vi "Keithley2400x2.vi"() -> ()   [LabVIEW 2014]
uses:
  <vilib>/Utility/file.llb/Write To Spreadsheet File (string).vi
panel:
  in  "stop":bool
  in  "Source Mode  (0: Voltage)":u16(ring) items=["Voltage", "Current"]
  in  "VISA resource name 2":refnum<visa-resource-name>
  in  "Serial Configuration":T1={"Baud Rate"=9600, "Parity"=0, "Data Bits"=8, "Stop Bits"=10, "Flow Control"=0} {"Flow Control" items=["None", "XON/XOFF", "RTS/CTS", "XON/XOFF & RTS/CTS", "DTR/DSR", "XON/XOFF & DTR/DSR"]; "Stop Bits" items=["1.0"=10, "1.5"=15, "2.0"=20]; "Data Bits" items=["7"=7, "8"=8]; "Parity" items=["None", "Odd", "Even", "Mark", "Space"]; "Baud Rate" items=["300"=300, "600"=600, "1200"=1200, "2400"=2400, "4800"=4800, "9600"=9600, "19200"=19200]}
  in  "Файл записи замеров":path
  in  "Ограничение":dbl format="%.2f"
  out "Замер":string
  in  "Выход":dbl
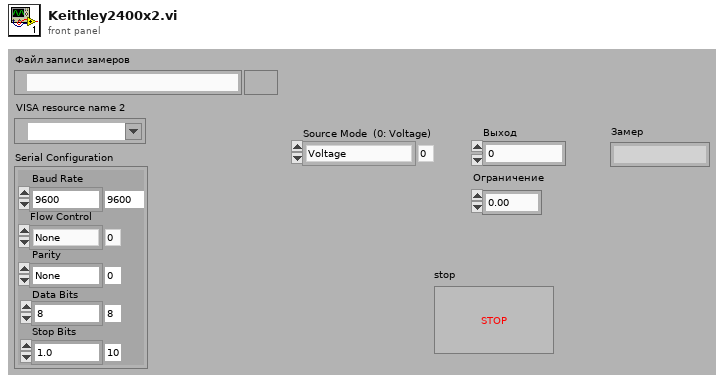
[diagram p1: front panel]
types:
  T1 = cluster{"Baud Rate":u32, "Parity":u16, "Data Bits":u16, "Stop Bits":u16, "Flow Control":u16}
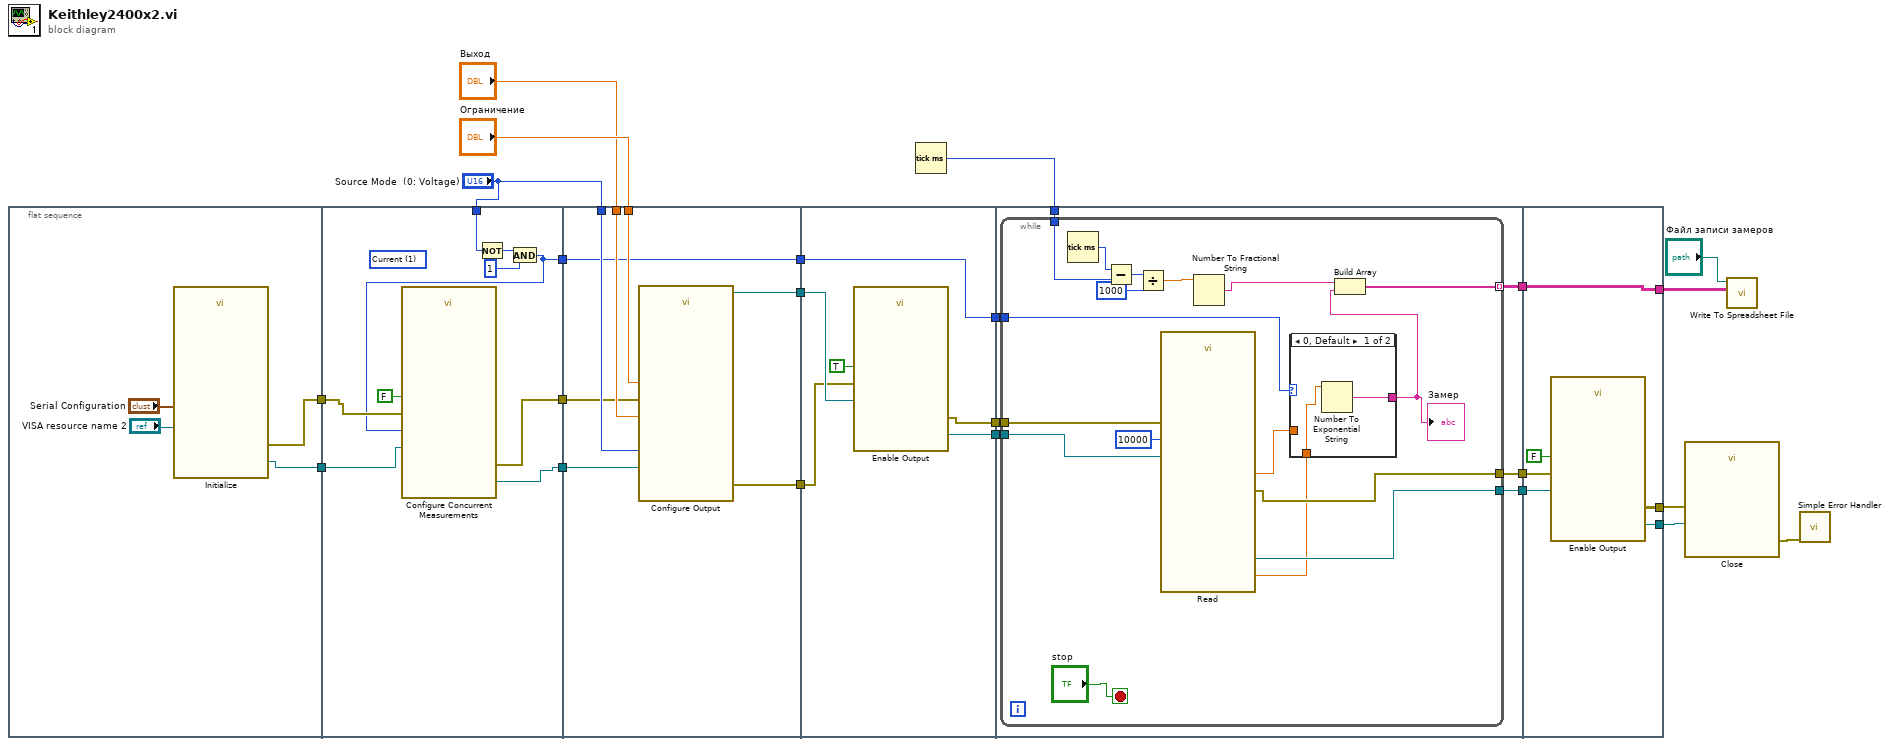
[diagram p0: block diagram]
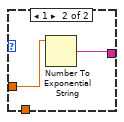
[diagram p2: hidden frame]
diagram:
  n1 = flat-sequence {
    tunnel: [w25] -> w8
    tunnel: [w24] -> w6
    tunnel: w8 -> [w34]
    tunnel: [w35] -> w7
    tunnel: w6 -> [w33]
    tunnel: [w36] -> w5
    tunnel: "Source Mode  (0: Voltage)" -> [w31]
    tunnel: [w28] -> w1
    tunnel: "Ограничение" -> [w44]
    tunnel: "Выход" -> [w43]
    tunnel: "Source Mode  (0: Voltage)" -> [w42]
    tunnel: w7 -> [w41]
    tunnel: w5 -> [w40]
    tunnel: [w39] -> w21
    tunnel: [w38] -> w20
    tunnel: [w37] -> w3
    tunnel: w1 -> [w37]
    tunnel: w21 -> [w50]
    tunnel: w20 -> [w49]
    tunnel: [w47] -> w19
    tunnel: [w46] -> w18
    tunnel: w3 -> [w45]
    tunnel: [w45] -> w2
    tunnel: w19 -> [w57]
    tunnel: w18 -> [w56]
    tunnel: w17 -> [w55]
    tunnel: [w54] -> w14
    tunnel: [w53] -> w13
    tunnel: [w52] -> w12
    tunnel: w2 -> [w51]
    tunnel: [w84] -> w15
    tunnel: w14 -> [w84]
    tunnel: w13 -> [w82]
    tunnel: w12 -> [w81]
    tunnel: [w80] -> w11
    tunnel: [w79] -> w10
    frame #0 {
      n2 = call "Initialize.vi"("Serial Configuration"="Serial Configuration", "VISA resource name"="VISA resource name 2") -> ("error out"=w24:errorcluster, "VISA resource name out"=w25:refnum<visa-resource-name>)  [unwired: 8 in]
    }
    frame #1 {
      (unwired) u16 1 items=["Volts", "Current", "Resistance", "Volt, Current", "Volts, Resistance", "Current, Resistance", "All"] ("Measurement Selection (3: Volts, Current)")
      n3 = Not(x=w31) -> (.not. x?=w30:u16)
      n4 = And(x=w30, y=u16 1) -> (x .and. y?=w28:u16)
      n5 = call "Configure Concurrent Measurements.vi"("error in (no error)"=w33, "Measurement Selection (3: Volts, Current)"=w28, "Enable Concurrent Measurements (F: Disable)"=FALSE, "VISA resource name"=w34) -> ("error out"=w36:errorcluster, "VISA resource name out"=w35:refnum<visa-resource-name>)  [unwired: 6 in]
    }
    frame #2 {
      n6 = call "Configure Output.vi"("Source Mode  (0: Voltage)"=w42, "error in (no error)"=w40, "Compliance  Level (0.1)"=w44, "Output Level (0)"=w43, "VISA resource name"=w41) -> ("error out"=w38:errorcluster, "VISA resource name out"=w39:refnum<visa-resource-name>)  [unwired: 5 in]
    }
    frame #3 {
      n7 = call "Enable Output.vi"("error in (no error)"=w49, "Enable Output (T: Enable)"=TRUE, "VISA resource name"=w50) -> ("error out"=w47:errorcluster, "VISA resource name out"=w46:refnum<visa-resource-name>)  [unwired: 7 in]
    }
    frame #4 {
      n8 = while {
        tunnel: w57 -> [w73]
        tunnel: w56 -> [w72]
        tunnel: w55 -> [w67]
        tunnel: [w62] -> w54 mode=indexing
        tunnel: [w65] -> w53
        tunnel: [w64] -> w52
        tunnel: w51 -> [w61]
        stop <- "stop" stop-if-true
        n9 = Tick Count (ms)() -> (millisecond timer value=w71:u32)
        n10 = Subtract(x=w71, y=w67) -> (x-y=w70:u32)
        n11 = Divide(x=w70, y=u32 1000) -> (x/y=w68:dbl)
        n12 = call-poly "Read.vi"("VISA resource name"=w72, "Timeout (10000 ms)"=10000, "error in (no error)"=w73) -> ("Voltage"=w59:sgl, "VISA resource name out"=w65:refnum<visa-resource-name>, "Current"=w60:sgl, "error out"=w64:errorcluster)  [unwired: 6 in, 3 out]
        n13 = Number To Fractional String(number=w68) -> (F-format string=w66:string)  [unwired: 3 in]
        n14 = case shown="0, Default" w61 {
          tunnel: w60 -> [_ w78]
          tunnel: w59 -> [w76 _]
          tunnel: [w75 w77] -> w58
          frame 0, Default {
            n15 = Number To Exponential String(number=w76) -> (E-format string=w75:string)  [unwired: 3 in]
          }
          frame 1 {
            n16 = Number To Exponential String(number=w78) -> (E-format string=w77:string)  [unwired: 3 in]
          }
        }
        "Замер" <- w58
        n17 = Build Array(w66, w58) -> (w62:string[])
      }
    }
    frame #5 {
      n18 = call "Enable Output.vi"("error in (no error)"=w81, "Enable Output (T: Enable)"=FALSE, "VISA resource name"=w82) -> ("error out"=w80:errorcluster, "VISA resource name out"=w79:refnum<visa-resource-name>)  [unwired: 7 in]
    }
  }
  n19 = Tick Count (ms)() -> (millisecond timer value=w17:u32)
  n20 = call "Close.vi"("error in (no error)"=w11, "VISA resource name"=w10) -> ("error out"=w9:errorcluster)  [unwired: 9 in]
  n21 = call-poly <vilib>:"Write To Spreadsheet File.vi"("2D data"=w15, "file path (dialog if empty)"="Файл записи замеров") -> ()  [unwired: 6 in, 1 out]
  n22 = call <vilib>:"Simple Error Handler.vi"("error in (no error)"=w9) -> ()  [unwired: 4 in, 5 out]
